vi "Launch QControl Creator.vi"(8 "error in (no error)":errorcluster, 11 "New QControl Info":refnum<data-value>) -> (0 "error out":errorcluster, 3 "CreatorRefnum":refnum<vi>)   [LabVIEW 2015, in "New QControl Info.lvclass"]
doc: "<b> </b> <b> </b>\n©2016 Q Software Innovations, LLC (QSI)\nwritten by Quentin Alldredge\nproduced in LabVIEW 2015\n\nsupport@qsoftwareinnovations.com\nwww.qsoftwareinnovations.com\n\nAll rights reserved.\n\nRedistribution and use in source and binary forms, with or without modification, are permitted provided that the following conditions are met:\n\n * Redistributions of source code must retain the above copyright notice, this list of conditions and the following disclaimer.\n * Redistributions in binary form must reproduce the above copyright notice, this list of conditions and the following disclaimer in the documentation and/or other materials provided with the distribution.\n * Neither the name of Q Software Innovations, LLC. nor the names of its contributors may be used to endorse or promote products derived from this software without specific prior written permission.\n\nTHIS SOFTWARE IS PROVIDED BY THE COPYRIGHT HOLDERS AND CONTRIBUTORS \"AS IS\" AND ANY EXPRESS OR IMPLIED WARRANTIES, INCLUDING, BUT NOT LIMITED TO, THE IMPLIED WARRANTIES OF MERCHANTABILITY AND FITNESS FOR A PARTICULAR PURPOSE ARE DISCLAIMED. IN NO EVENT SHALL THE COPYRIGHT OWNER OR CONTRIBUTORS BE LIABLE FOR ANY DIRECT, INDIRECT, INCIDENTAL, SPECIAL, EXEMPLARY, OR CONSEQUENTIAL DAMAGES (INCLUDING, BUT NOT LIMITED TO, PROCUREMENT OF SUBSTITUTE GOODS OR SERVICES; LOSS OF USE, DATA, OR PROFITS; OR BUSINESS INTERRUPTION) HOWEVER CAUSED AND ON ANY THEORY OF LIABILITY, WHETHER IN CONTRACT, STRICT LIABILITY, OR TORT (INCLUDING NEGLIGENCE OR OTHERWISE) ARISING IN ANY WAY OUT OF THE USE OF THIS SOFTWARE, EVEN IF ADVISED OF THE POSSIBILITY OF SUCH DAMAGE."
uses:
  New QControl Info.lvclass
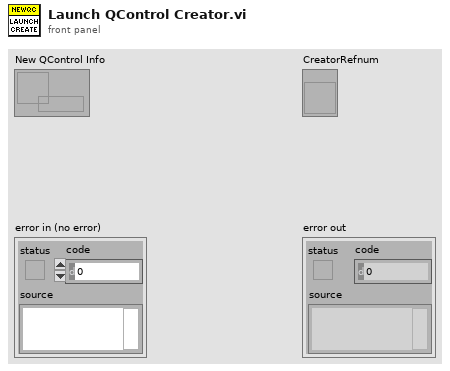
[diagram p1: front panel]
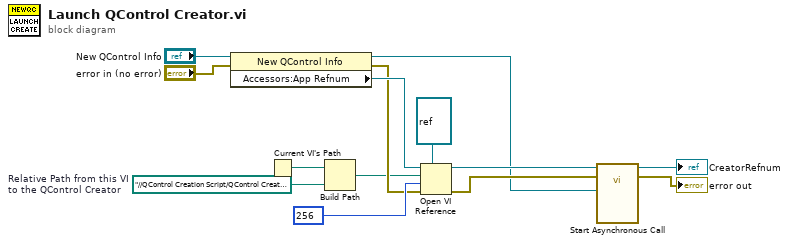
[diagram p0: block diagram]
diagram:
  w3 = path "../../QControl Creation Script/QControl Creator Core.vi"  # Relative Path from this VI to the QControl Creator
  n1 = property class="New QControl Info"(reference="New QControl Info", error in="error in (no error)") -> (reference out=w7:refnum<data-value>, error out=w5:errorcluster, "Accessors:App Refnum"=w9:refnum<vi>)
  n2 = Current VI's Path() -> (path=w4:path)
  n3 = Build Path(base path=w4, name or relative path=w3) -> (appended path=w2:path)
  n4 = Open VI Reference(type specifier VI Refnum (for type only)=refnum<vi> refnum, application reference (local)=w9, vi path=w2, options=256, error in (no error)=w5) -> (vi reference=w13:refnum<vi>, error out=w10:errorcluster)  [unwired: 1 in]
  n5 = call-by-ref "Start Asynchronous Call"(reference=w13, error in=w10, "New QControl Info"=w7) -> (reference out=→"CreatorRefnum":refnum<vi>, error out=→"error out":errorcluster)  [unwired: 10 in, 1 out]
